vi "Billede_1_modtag.vi"() -> ()   [LabVIEW 2018]
uses:
  <vilib>/myRIO/Instrument Drivers/Onboard IO/UART/typedef/VISA Configuration.ctl
  <vilib>/Instr/_visa.llb/VISA Configure Serial Port (Instr).vi
  <vilib>/myRIO/Express VI/Onboard IO/UART/UART Express VI.xnode
  <vilib>/myRIO/Instrument Drivers/Onboard IO/UART/UART.lvlib
panel:
  out "length":i32
  out "Characters Read":string
  in  "stop":bool
  out "Intensity Graph 4":u8[][](graph)
  out "array":u8[][](array[numeric])
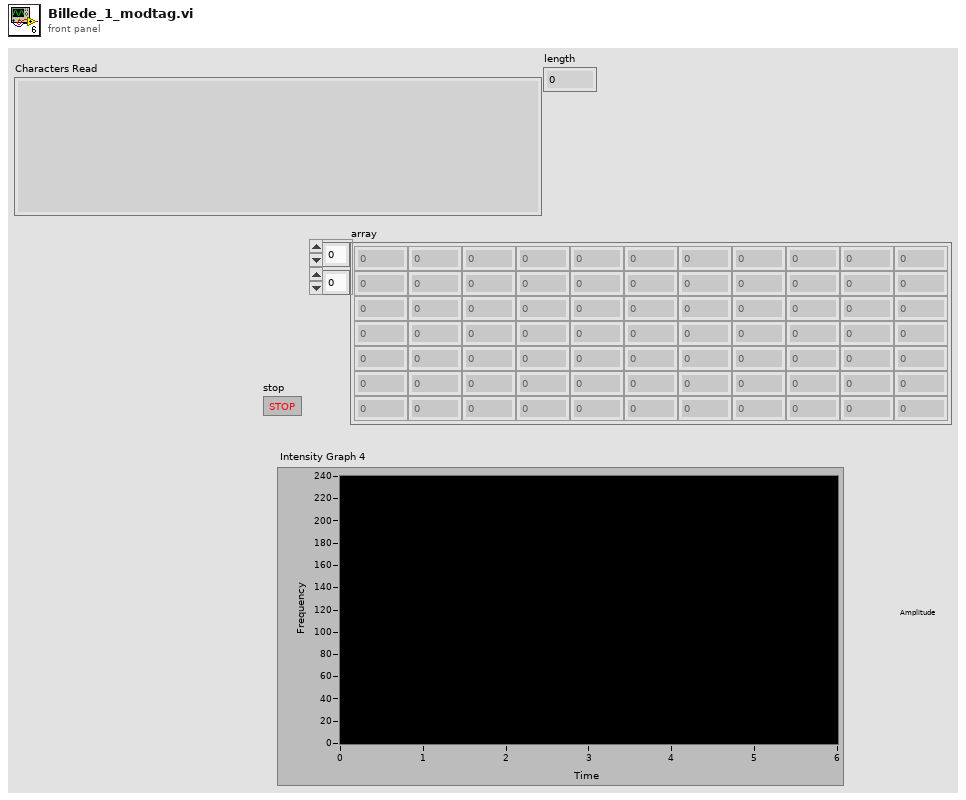
[diagram p1: front panel]
types:
  T1 = typedef "UART.lvlib/VISA Configuration.ctl" = cluster{"baud rate (9600)":u32, "data bits (8)":u16, "parity (0:none)":enum16{"None", "Odd", "Even", "Mark", "Space"}, "stop bits (10: 1 bit)":u16, "flow control (0:none)":u16, "termination char\n(0xA = '\\n' = LF) ":u8, "Enable Termination\nChar (T)":bool, "timeout (10sec)":u32}
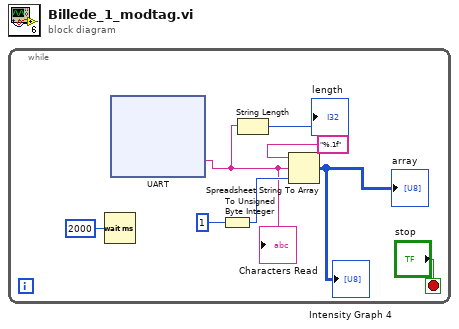
[diagram p0: block diagram]
diagram:
  n1 = while {
    stop <- "stop" stop-if-true
    n2 = Wait (ms)(milliseconds to wait=u32 2000) -> ()  [unwired: 1 out]
    n3 = xnode "UART"() -> ("Characters Read"=w3:string)  [unwired: 1 in, 1 out]
    "Characters Read" <- w3
    n4 = To Unsigned Byte Integer(number=u8 1) -> (unsigned 8bit integer=w7:u8)
    n5 = String Length(string=w3) -> (length=→"length":i32)
    n6 = Spreadsheet String To Array(format string="%.1f", spreadsheet string=w3, array type (2D Dbl)=w7) -> (array=→"array" →"Intensity Graph 4":u8[][])  [unwired: 1 in]
  }
